vi "Get MDIF Blocks (All).vi"(8 "error in (no error)":errorcluster, 11 "MDIF reference in":refnum<k24>) -> (0 "error out":errorcluster, 2 "MDIF Blocks":T1[](array[typedef]), 3 "MDIF reference out":refnum<k24>)   [LabVIEW 2023, in "NI_HFNetworkAnalysis.lvlib"]
doc: "Retrieve all the MDIF blocks in memory for the referenced MDIF file."
uses:
  NI_HFNetworkAnalysis.lvlib
  C:/srd-semi-rfcal-software/AuxTools/STSRFFixtureCharactUtility/Source/Code Modules/Fixture/Dependencies/HFNetworkAnalysis/Support Files/NACE.Utils.Data.dll
  Support Files/NACE.Utils.Data.dll
  Controls/MDIF Block.ctl
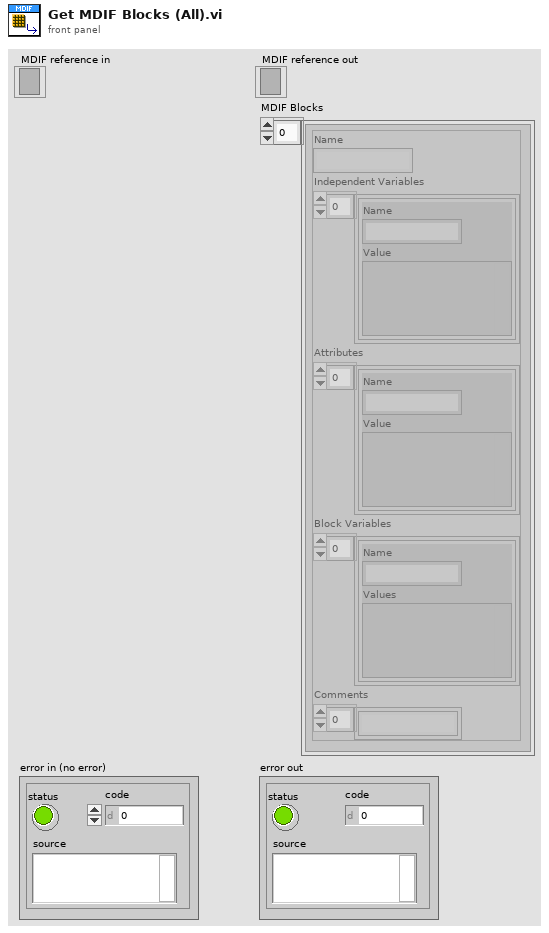
[diagram p1: front panel]
types:
  T1 = typedef "NI_HFNetworkAnalysis.lvlib/MDIF Block.ctl" = cluster{"Name":string, "Independent Variables":cluster{"Name":string, "Value":variant}[], "Attributes":cluster{"Name":string, "Value":variant}[], "Block Variables":cluster{"Name":string, "Values":variant}[], "Comments":string[]}
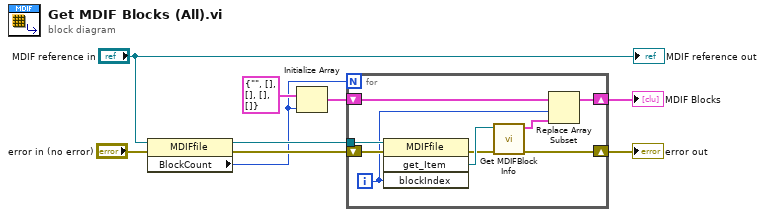
[diagram p0: block diagram]
diagram:
  n1 = property class="MDIFfile"(reference="MDIF reference in", error in="error in (no error)") -> (reference out=w9:refnum<k24>, error out=w8:errorcluster, "BlockCount"=w3:i32)
  n2 = Initialize Array(T1 {"Name"="", "Independent Variables"=[], "Attributes"=[], "Block Variables"=[], "Comments"=[]} ("MDIF Block"), w3) -> (w2:T1[])
  n3 = for {
    N: w3 -> [_]
    tunnel: w9 -> [w18]
    shift-right: [w15] -> w5
    shift-left: w8 -> [w16]
    shift-right: [w12] -> w1
    shift-left: w2 -> [w13]
    i -> [w10]
    n4 = invoke class="MDIFfile" method="get_Item"(reference=w18, error in=w16, "blockIndex"=w10) -> (error out=w14:errorcluster, "get_Item"=w17:refnum<k24>)  [unwired: 1 in, 2 out]
    n5 = call "Get MDIFBlock Info.vi"("error in (no error)"=w14, "MDIF Block Refnum in"=w17) -> ("error out"=w15:errorcluster, "MDIF Block"=w11:T1)  [unwired: 8 in]
    n6 = Replace Array Subset(array=w13, new element=w11, index=w10) -> (w12:T1[])
  }
  "MDIF Blocks" <- w1
  "error out" <- w5
  "MDIF reference out" <- "MDIF reference in"
